vi "Main.vi"   [LabVIEW 2013]
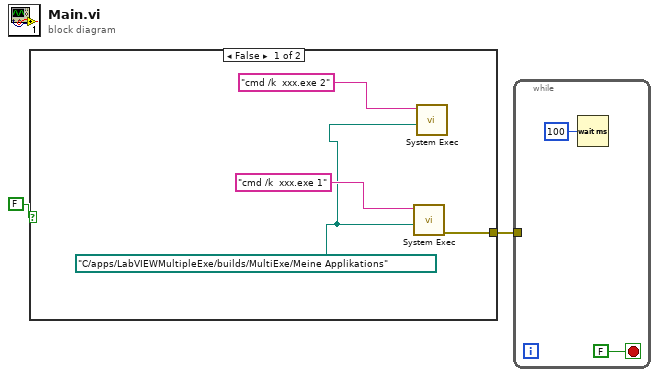
[diagram p0: block diagram]
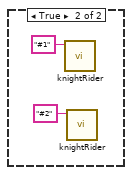
[diagram p2: hidden frame]
diagram:
  n1 = case shown="False" FALSE {
    tunnel: [w5 _] -> w1
    frame False {
      w3 = path "C:/apps/LabVIEWMultipleExe/builds/MultiExe/Meine Applikations" ("working directory")
      n2 = call <vilib>:"System Exec.vi"("working directory"=w3, "command line"="cmd /k  xxx.exe 1") -> ("error out"=w5:errorcluster)  [unwired: 6 in, 3 out]
      n3 = call <vilib>:"System Exec.vi"("working directory"=w3, "command line"="cmd /k  xxx.exe 2") -> ()  [unwired: 6 in, 4 out]
    }
    frame True {
      n4 = call "knightRider.vi"("String"="#1") -> ()  [unwired: 10 in]
      n5 = call "knightRider.vi"("String"="#2") -> ()  [unwired: 10 in]
    }
  }
  n6 = while {
    tunnel: w1 -> [_]
    stop <- FALSE stop-if-true
    n7 = Wait (ms)(milliseconds to wait=u32 100 ("Zu wartende ms")) -> ()  [unwired: 1 out]
  }
